vi "7L22-Qs_Poisson_Gauss.vi"(5 "err in":errorcluster caption="entrée d'erreur (pas d'erreur)", 8 "Qs (e)":T2, 9 "Histo (e)":T1) -> (2 "Qs (s)":T2, 3 "Histo (s)":T1, 4 "err out":errorcluster caption="sortie d'erreur")   [LabVIEW 2010, in "lv_07.lvlib"]
doc: "En fonction du délai d d'approvisionnement, du risque de rupture (5% par défaut) et des données d'historique, le VI calcule le seuil minimum de réapprovisionnement Qs selon les modèles de Poisson et de Gauss."
uses:
  lv_07.lvlib
  c_histo.ctl
  c_Qs_.ctl
  lv_02/5-k-invdist.vi
  lv_02/lv_02.lvlib
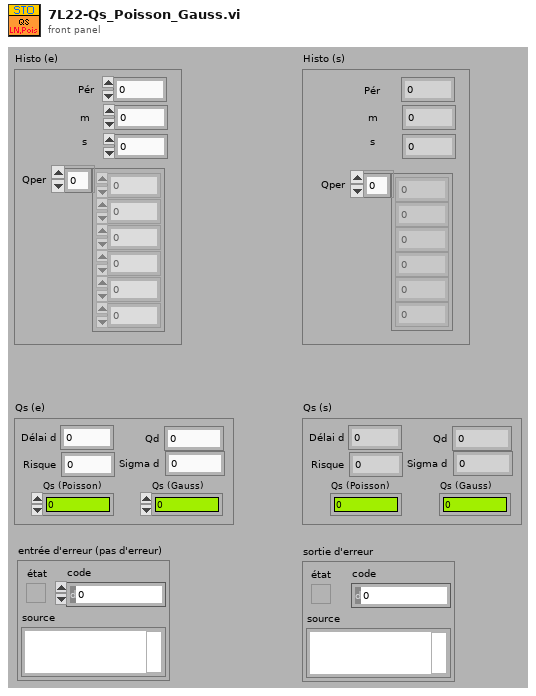
[diagram p1: front panel]
types:
  T1 = typedef "lv_07.lvlib/c_histo.ctl" = cluster{"Pér":dbl, "Qper":dbl[], "s":dbl, "m":dbl}
  T2 = typedef "lv_07.lvlib/c_Qs_.ctl" = cluster{"Sigma d":dbl, "Qs (Gauss)":dbl, "Qs (Poisson)":dbl, "Qd":dbl, "Délai d":dbl, "Risque":dbl}
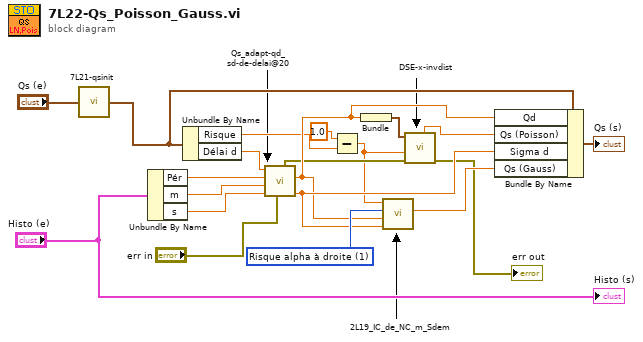
[diagram p0: block diagram]
diagram:
  w15 = u16 1 items=["Risque alpha bilattéral", "Risque alpha à droite", "Risque alpha à gauche"] ("Niveau de confiance")
  n1 = call "7L21-qsinit.vi"("Qs (e)"="Qs (e)") -> ("Qs (s)"=w8:T2)
  n2 = Unbundle By Name("Histo (e)") -> ("Pér"=w19:dbl, "m"=w17:dbl, "s"=w18:dbl)
  n3 = Unbundle By Name(w8) -> ("Risque"=w5:dbl, "Délai d"=w12:dbl)
  n4 = call "Qs_adapt-qd_sd-de-delai@20.vi"("error in (no error)"="err in", "Sigma"=w18, "Moyenne"=w17, "Durée"=w19, "Délai d"=w12) -> ("Sigma d"=w13:dbl, "Qd"=w7:dbl, "error out"=w3:errorcluster)  [unwired: 2 in]
  n5 = Subtract(x=1.0 ("y"), y=w5) -> (x-y=w1:dbl)
  n6 = Bundle("Qd"=w7) -> (w6:cluster{"Qd":dbl})  [unwired: 1 in]
  n7 = call "2L19_IC_de_NC_m_Sdem.vi"("S dem"=w13, "m"=w7, "Niveau de confiance"=w15, "NC"=w1) -> ("Ic max"=w14:dbl)  [unwired: 6 in, 1 out]
  n8 = call-poly "DSE-x-invdist.vi"("err in"=w3, "F(k)"=w1, "Loi de Poisson"=w6) -> ("err out"=→"err out":errorcluster, "k interpolé"=w4:dbl)  [unwired: 4 in, 3 out]
  n9 = Bundle By Name(cluster=w8, "Qd"=w7, "Qs (Poisson)"=w4, "Sigma d"=w13, "Qs (Gauss)"=w14) -> (→"Qs (s)":T2)
  "Histo (s)" <- "Histo (e)"
